vi "TurnCrank.vi"(8 "error in (no error)":errorcluster, 11 "object in":refnum<class "HasMoneyState.lvclass">) -> (0 "error out":errorcluster, 3 "object out":refnum<class "State.lvclass">)   [LabVIEW 2020, in "HasMoneyState.lvclass"]
uses:
  HasMoneyState.lvclass
  C:/Projects/OpenGDS_DesignPatterns/State1/State_class/State.lvclass
  State_class/State.lvclass
  SoldState_class/SoldState.lvclass
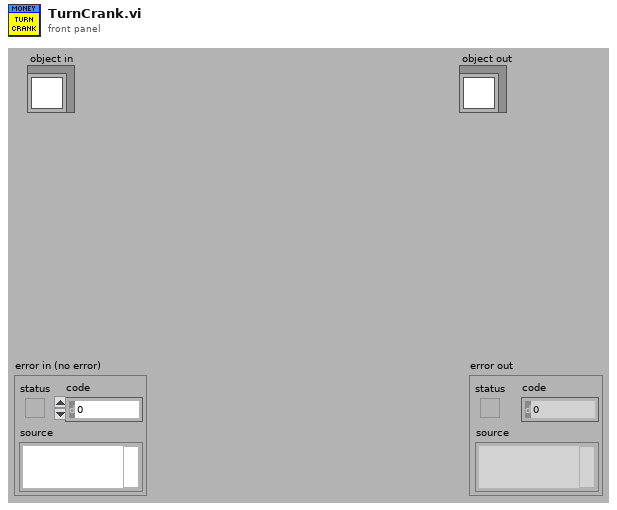
[diagram p1: front panel]
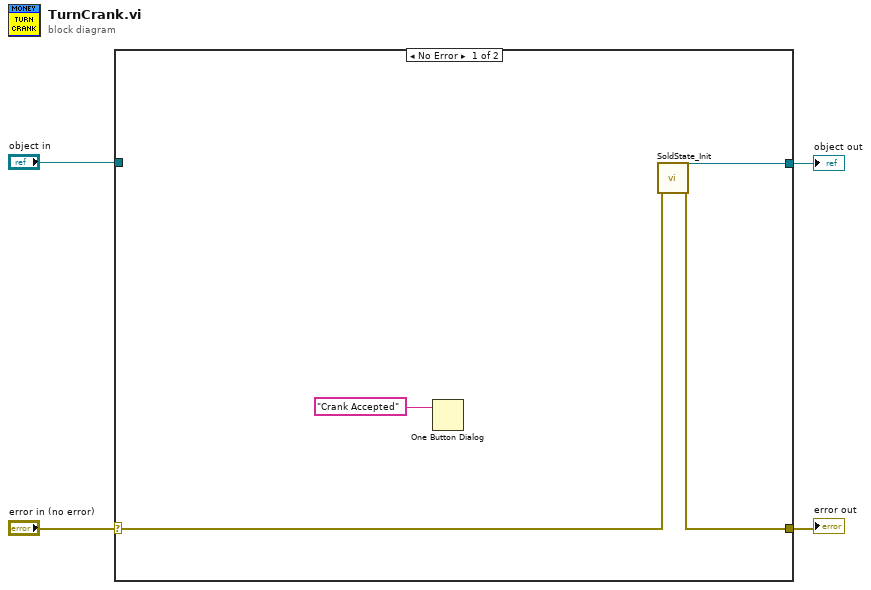
[diagram p0: block diagram]
diagram:
  n1 = case shown="No Error" "error in (no error)" {
    selector: "error in (no error)" -> [w7 w10]
    tunnel: [w6 w10] -> w3
    tunnel: [w8 w9] -> w1
    tunnel: "object in" -> [_ w9]
    frame No Error {
      n2 = One Button Dialog(message="Crank Accepted" ("TextIn")) -> ()  [unwired: 1 in, 1 out]
      n3 = call "SoldState_Init.vi"("error in (no error)"=w7) -> ("error out"=w6:errorcluster, "object out"=w8:refnum<class "SoldState.lvclass">)  [unwired: 9 in]
    }
    frame Error {
    }
  }
  "error out" <- w3
  "object out" <- w1
